vi "Close Ref.vi"(8 "error in (no error)":errorcluster, 11 "Serial Device in":refnum<class "Serial Device.lvclass">) -> (0 "error out":errorcluster, 3 "Serial Device out":refnum<class "Serial Device.lvclass">)   [LabVIEW 2016, in "Serial Hardware.lvlib" / "Serial Device.lvclass"]
uses:
  Serial Device.lvclass
  Serial Device.lvclass/Serial Device.ctl
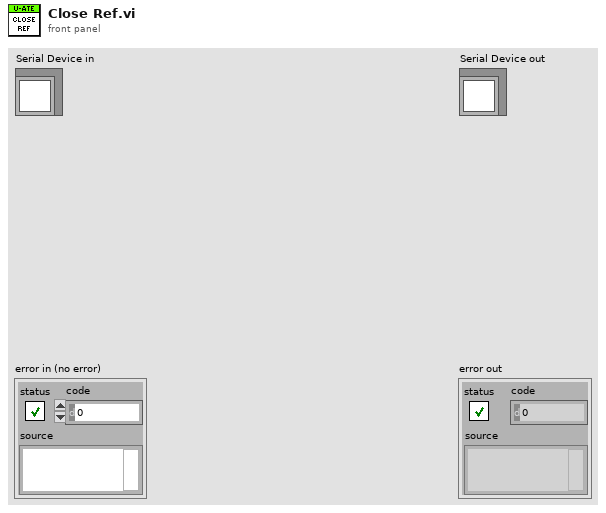
[diagram p1: front panel]
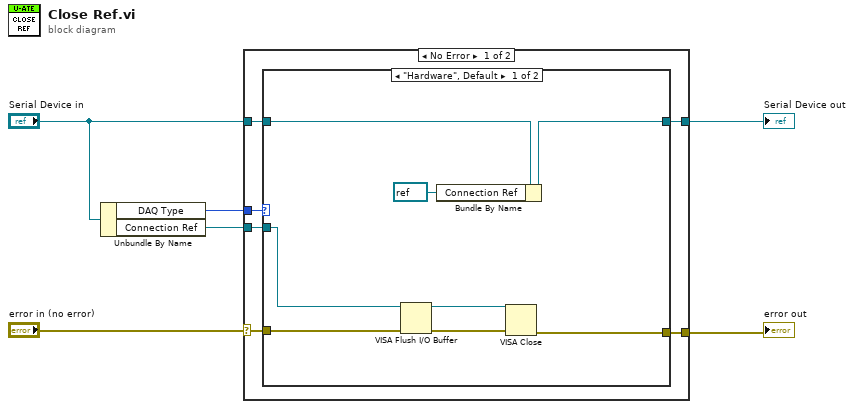
[diagram p0: block diagram]
diagram:
  n1 = Unbundle By Name("Serial Device in") -> ("DAQ Type"=w4:enum16{"Hardware", "Simulation"}, "Connection Ref"=w3:refnum<visa-resource-name>)
  n2 = case shown="No Error" "error in (no error)" {
    selector: "error in (no error)" -> [w10 w23]
    tunnel: "Serial Device in" -> [w8 w24]
    tunnel: w4 -> [w12 _]
    tunnel: w3 -> [w11 _]
    tunnel: [w9 w23] -> w2
    tunnel: [w7 w24] -> w1
    frame No Error {
      n3 = case shown="\"Hardware\", Default" w12 {
        tunnel: w11 -> [w19 _]
        tunnel: w10 -> [w20 w21]
        tunnel: [w16 w21] -> w9
        tunnel: w8 -> [w15 w22]
        tunnel: [w14 w22] -> w7
        frame "Hardware", Default {
          n4 = VISA Flush I/O Buffer(VISA resource name=w19, error in (no error)=w20) -> (VISA resource name out=w18:refnum<visa-resource-name>, error out=w17:errorcluster)  [unwired: 1 in]
          n5 = Bundle By Name(cluster=w15, "Connection Ref"=refnum<visa-resource-name> refnum) -> (w14:refnum<class "Serial Device.lvclass">)
          n6 = VISA Close(VISA resource name=w18, error in (no error)=w17) -> (error out=w16:errorcluster)
        }
        frame "Simulation" {
        }
      }
    }
    frame Error {
    }
  }
  "error out" <- w2
  "Serial Device out" <- w1
